vi "FPGA_Amplitude_Pockels_Galvo.vi"(5 "Live(F)/Functional(T)":bool, 6 "Chirp index":i32, 7 "FPGA Type":enum16{"Virtex 5", "Virtex 7"}(ring), 9 "difftime - aodcontrol delay":dbl, 10 "Laser(V) - Vertex 7 Only":dbl[](array[numeric]), 11 "Amplitude":dbl[](array[numeric])) -> (2 "Pockels_Galvo_Params":T1)   [LabVIEW 2017]
uses:
  Controls/Pockels_Galvo_Params.ctl
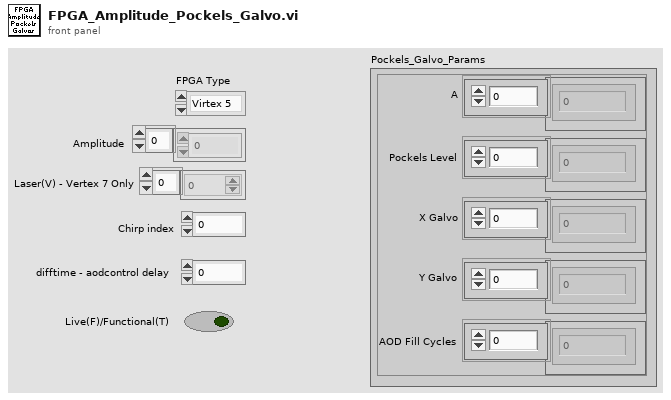
[diagram p1: front panel]
types:
  T1 = typedef "Pockels_Galvo_Params.ctl" = cluster{"A":dbl[], "Pockels Level":dbl[], "X Galvo":dbl[], "Y Galvo":dbl[], "AOD Fill Cycles":dbl[]}
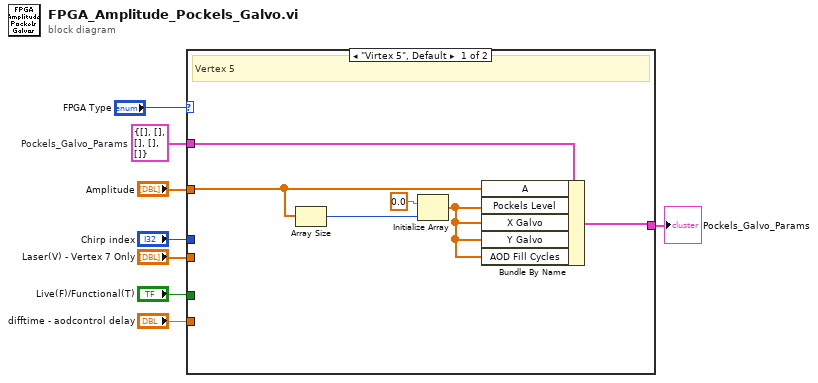
[diagram p0: block diagram]
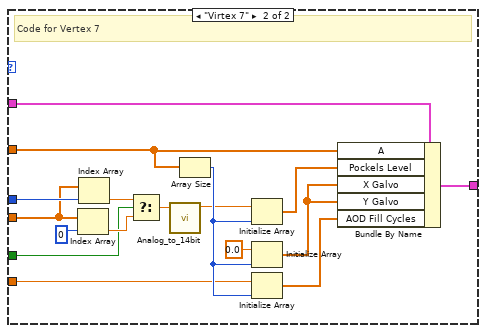
[diagram p2: hidden frame]
diagram:
  w8 = T1 {"A"=[], "Pockels Level"=[], "X Galvo"=[], "Y Galvo"=[], "AOD Fill Cycles"=[]}  # Pockels_Galvo_Params
  n1 = case shown="\"Virtex 5\", Default" "FPGA Type" {
    tunnel: w8 -> [w13 w22]
    tunnel: "Amplitude" -> [w10 w21]
    tunnel: "Chirp index" -> [_ w20]
    tunnel: "Laser(V) - Vertex 7 Only" -> [_ w19]
    tunnel: "difftime - aodcontrol delay" -> [_ w17]
    tunnel: "Live(F)/Functional(T)" -> [_ w16]
    tunnel: [w14 w15] -> w2
    frame "Virtex 5", Default {
      # "Vertex 5"
      n2 = Array Size(array=w10) -> (size(s)=w11:i32)
      n3 = Initialize Array(0.0 ("element"), w11) -> (w9:dbl[])
      n4 = Bundle By Name(cluster=w13, "A"=w10, "Pockels Level"=w9, "X Galvo"=w9, "Y Galvo"=w9, "AOD Fill Cycles"=w9) -> (w14:T1)
    }
    frame "Virtex 7" {
      # "Code for Vertex 7"
      n5 = Index Array(array=w19, index=0) -> (element=w23:dbl)
      n6 = Index Array(array=w19, index=w20) -> (element=w24:dbl)
      n7 = Select(t=w24, s=w16, f=w23) -> (s? t:f=w25:dbl)
      n8 = call "Analog_to_14bit.vi"("Pockels (0-2V)"=w25) -> ("Pockels Level(14 bit)"=w26:dbl)  [unwired: 10 in]
      n9 = Array Size(array=w21) -> (size(s)=w27:i32)
      n10 = Initialize Array(w26, w27) -> (w28:dbl[])
      n11 = Initialize Array(0.0 ("element"), w27) -> (w31:dbl[])
      n12 = Initialize Array(w17, w27) -> (w30:dbl[])
      n13 = Bundle By Name(cluster=w22, "A"=w21, "Pockels Level"=w28, "X Galvo"=w31, "Y Galvo"=w31, "AOD Fill Cycles"=w30) -> (w15:T1)
    }
  }
  "Pockels_Galvo_Params" <- w2
